vi "acquireAndDetectTest.vi"() -> ()   [LabVIEW 2024]
uses:
  elements/black-squircle-dropdown.ctl
  toolkit/modelParameters.ctl
  elements/black-squircle-ring.ctl
  <vilib>/userDefined/High Color/IMAQdx.ctl
  <vilib>/Utility/error.llb/DialogType.ctl
  <vilib>/vision/driver/NI_Vision_Acquisition_Software.lvlib
  <resource>/objmgr/imaqdx.rc
  toolkit/transformCv.lvclass
panel:
  out "error status":string
  in  "update model":bool
  in  "res":T1 caption="Resolution:" items=["160x120 YUY2 30.00fps", "320x180 YUY2 30.00fps", "320x240 YUY2 30.00fps", "424x240 YUY2 30.00fps", "640x360 MJPG 30.00fps", "640x360 YUY2 30.00fps", "640x480 MJPG 30.00fps", "640x480 YUY2 30.00fps", "848x480 MJPG 30.00fps", "960x540 MJPG 30.00fps", "1280x720 MJPG 30.00fps"]
  in  "pause":bool
  in  "model params":T2={"conf"=0.25, "iou"=0.5, "model w"=1280, "model h"=736, "img w "=1280, "img h"=736} caption="Model Parameters"
  in  "classes":path caption="Class Definition Path"
  in  "model":path caption="Model Path"
  in  "cpu/gpu":enum32{"Item 0", "Item 1"}(radio)=enum."Item 1"
  in  "play":bool
  in  "cam":T3 caption="Camera:"
  out "img":T4(plugin-control)
  out "tot detect":i32 caption="Total Detections"
  # "Transform-CV Acquire and Detect Demo v1.0.0"
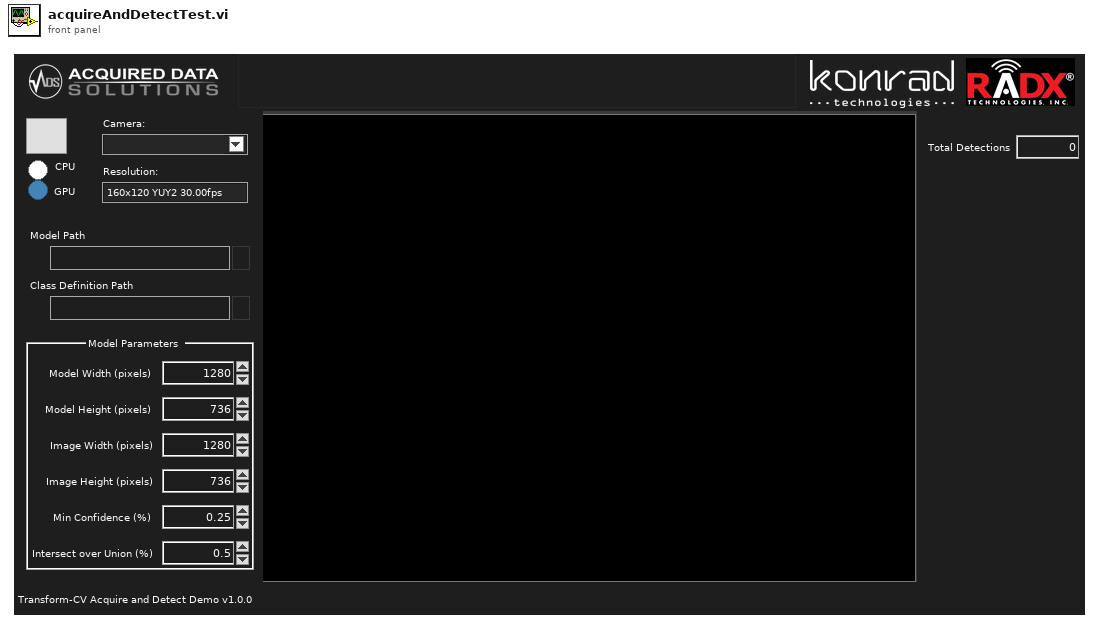
[diagram p1: front panel]
types:
  T1 = typedef "black-squircle-ring.ctl" = u16
  T2 = typedef "transformCv.lvclass/modelParameters.ctl" = cluster{"conf":dbl, "iou":dbl, "model w":i32, "model h":i32, "img w ":i32, "img h":i32}
  T3 = typedef "black-squircle-dropdown.ctl" = string
  T4 = typedef "IMAQ Image.ctl" = refnum<image>
  T5 = typedef "IMAQdx.ctl" = refnum<k21>
  T6 = cluster{"Left":i32, "Top":i32, "Right":i32, "Bottom":i32}
  T7 = typedef "transformCv.lvclass/rectangularDetectedObject.ctl" = cluster{"x1":sgl, "y1":sgl, "x2":sgl, "y2":sgl, "conf":sgl, "cls":i32}
  T8 = typedef "DialogType.ctl" = u16
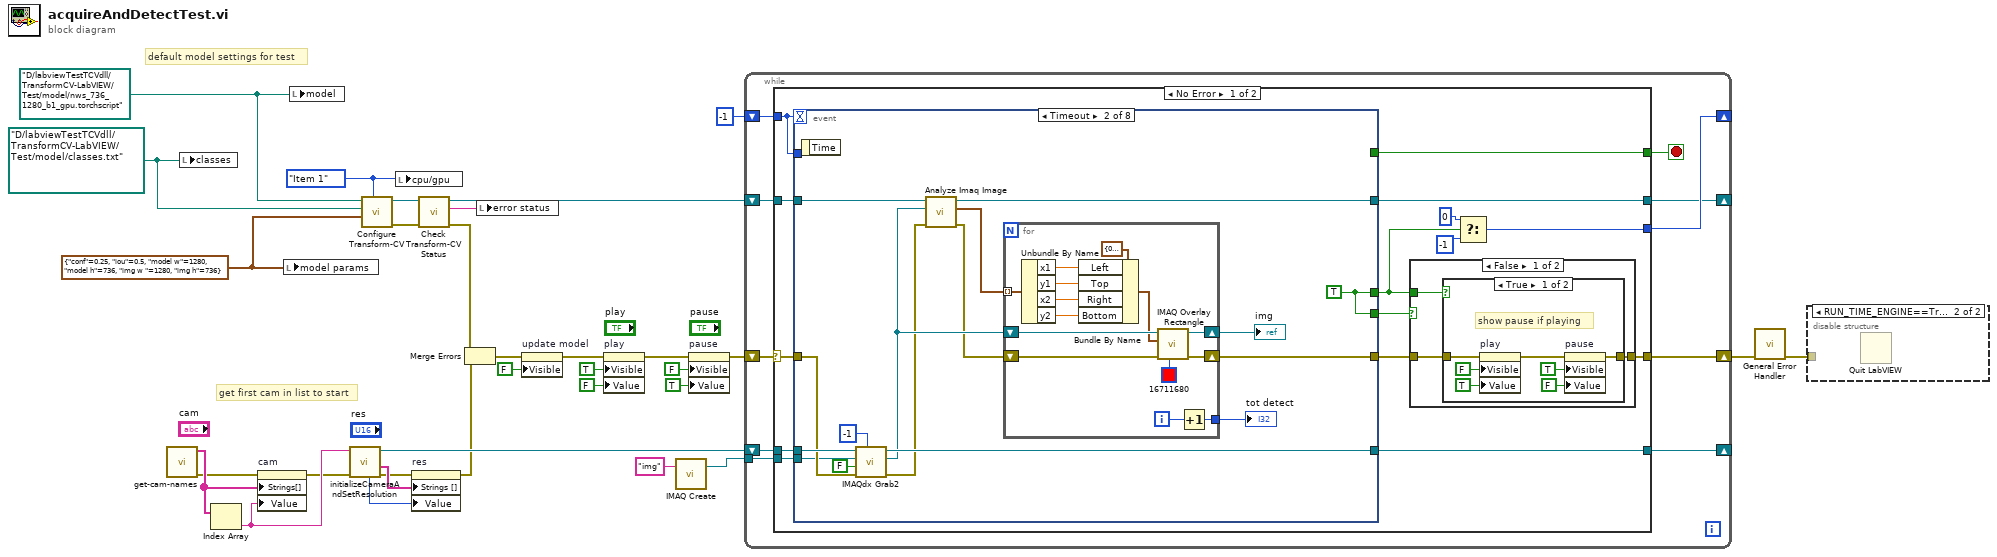
[diagram p0: block diagram]
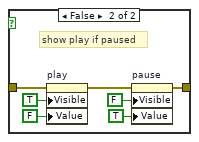
[diagram p3: hidden frame]
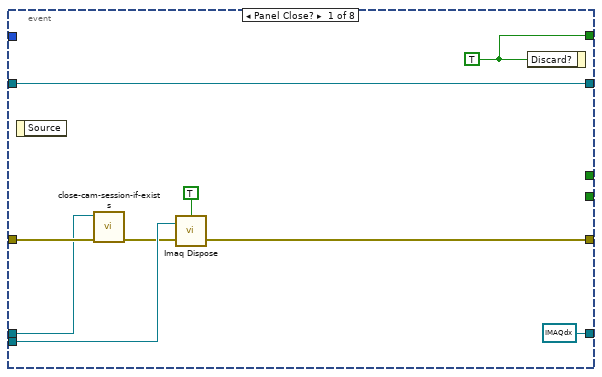
[diagram p5: hidden frame]
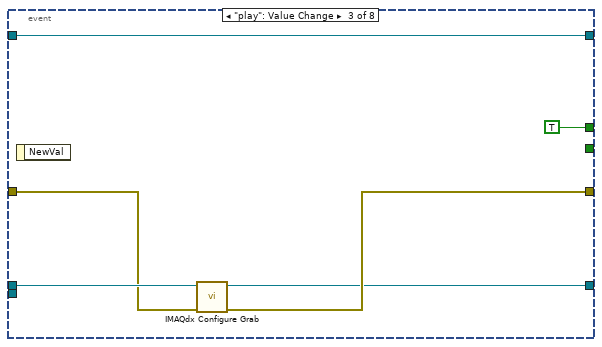
[diagram p6: hidden frame]
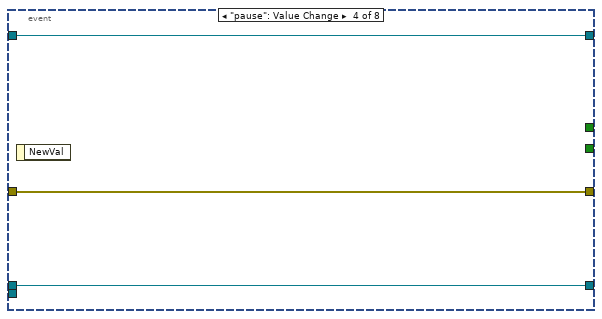
[diagram p7: hidden frame]
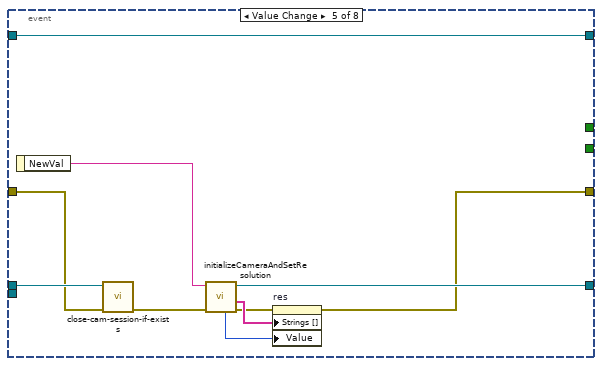
[diagram p8: hidden frame]
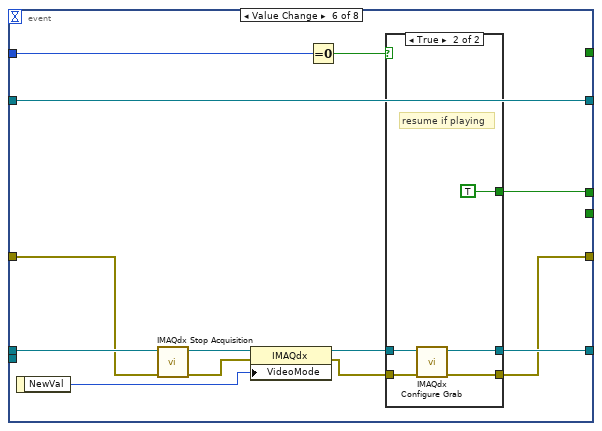
[diagram p9: hidden frame]
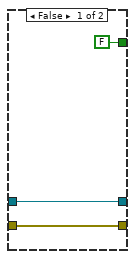
[diagram p10: hidden frame]
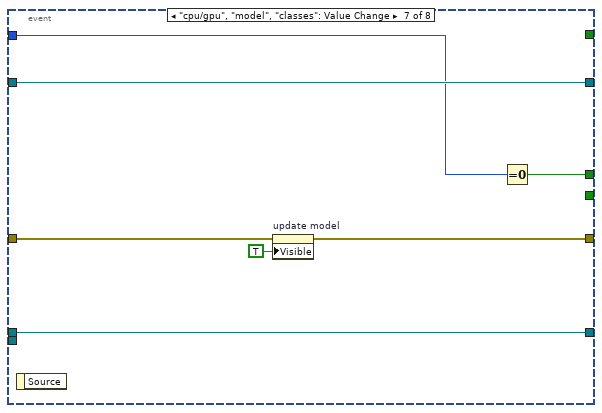
[diagram p11: hidden frame]
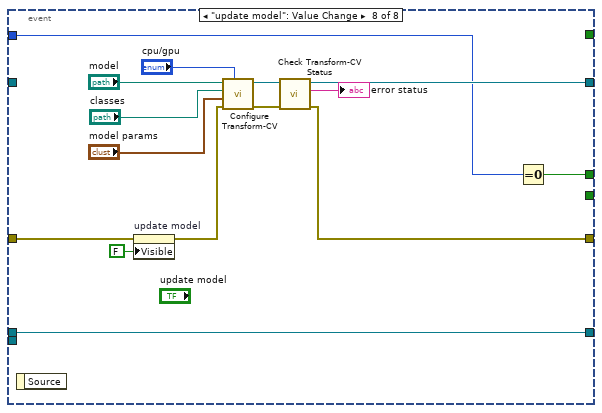
[diagram p12: hidden frame]
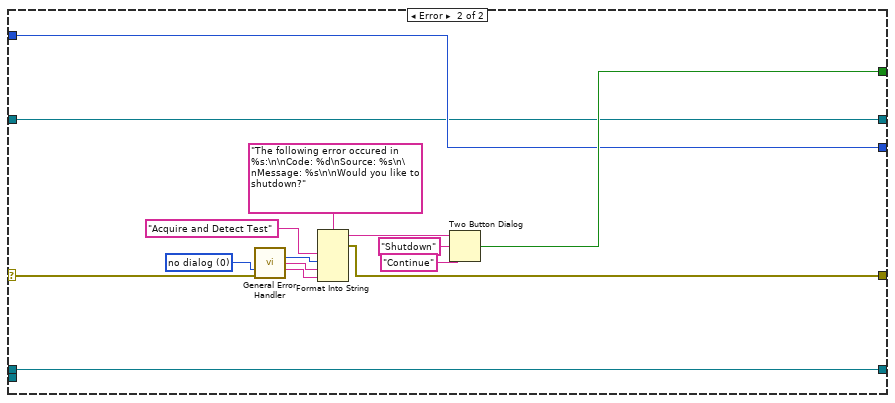
[diagram p13: hidden frame]
diagram:
  w8 = enum32{"Item 0", "Item 1"}."Item 1" ("cpu/gpu")
  w11 = T2 {"conf"=0.25, "iou"=0.5, "model w"=1280, "model h"=736, "img w "=1280, "img h"=736} ("model params")
  w12 = path "D:/labviewTestTCVdll/TransformCV-LabVIEW/Test/model/classes.txt" ("model")
  w13 = path "D:/labviewTestTCVdll/TransformCV-LabVIEW/Test/model/nws_736_1280_b1_gpu.torchscript" ("model")
  # "get first cam in list to start"
  # "default model settings for test"
  n1 = call "get-cam-names.vi"() -> ("error out"=w14:errorcluster, "cam names"=w25:string[])  [unwired: 10 in]
  n2 = local write "classes"(w12) -> ()
  n3 = Index Array(array=w25) -> (element=w24:string)  [unwired: 1 in]
  n4 = property on="cam" class="CmbBox (strict)"(error in=w14, "Strings[]"=w25, "Value"=w24) -> (error out=w23:errorcluster)  [unwired: 1 in, 1 out]
  n5 = local write "model params"(w11) -> ()
  n6 = local write "model"(w13) -> ()
  n7 = call "initializeCameraAndSetResolution.vi"("error in"=w23, "seesion in"=w24) -> ("error out"=w20:errorcluster, "mode names"=w22:string[], "session out"=w19:T5, "current mode"=w21:u32)  [unwired: 5 in, 1 out]
  n8 = call "Configure Transform-CV.vi"("cpu/gpu"=w8, "model params"=w11, "classes"=w12, "model"=w13) -> ("error out"=w6:errorcluster, "transformCvToolkit out"=w7:refnum<class "transformCv.lvclass">)  [unwired: 5 in, 1 out]
  n9 = local write "cpu/gpu"(w8) -> ()
  n10 = property on="res" class="Ring (strict)"(error in=w20, "Strings []"=w22, "Value"=w21) -> (error out=w10:errorcluster)  [unwired: 1 in, 1 out]
  n11 = call "Check Transform-CV Status.vi"("error in (no error)"=w6, "transformCv in"=w7) -> ("error out"=w5:errorcluster, "status"=w3:string, "transformCv out"=w4:refnum<class "transformCv.lvclass">)  [unwired: 7 in]
  n12 = Merge Errors(w5, w10) -> (w9:errorcluster)
  n13 = local write "error status"(w3) -> ()
  n14 = property on="update model" class="Bool"(error in=w9, "Visible"=FALSE) -> (error out=w16:errorcluster)  [unwired: 1 in, 1 out]
  n15 = property on="play" class="Bool (strict)"(error in=w16, "Visible"=TRUE, "Value"=FALSE ("play")) -> (error out=w30:errorcluster)  [unwired: 1 in, 1 out]
  n16 = call "IMAQ Create"("Image Name"="img") -> ("New Image"=w17:T4)  [unwired: 4 in, 1 out]
  n17 = property on="pause" class="Bool (strict)"(error in=w30, "Visible"=FALSE, "Value"=TRUE ("Visible")) -> (error out=w31:errorcluster)  [unwired: 1 in, 1 out]
  n18 = while {
    shift-right: [w42] -> w2
    shift-left: w31 -> [w41]
    shift-right: [w38] -> _
    shift-left: -1 -> [w39]
    shift-right: [w36] -> _
    shift-left: w19 -> [w37]
    tunnel: w17 -> [w35]
    shift-right: [w33] -> _
    shift-left: w4 -> [w34]
    stop <- w40 stop-if-true
    n19 = case shown="No Error" w41 {
      selector: w41 -> [w57 w183]
      tunnel: [w51 w181] -> w42
      tunnel: [w56 w182] -> w40
      tunnel: w39 -> [w45 w179]
      tunnel: [w53 w179] -> w38
      tunnel: w37 -> [w48 w178]
      tunnel: [w47 w178] -> w36
      tunnel: w35 -> [w46 _]
      tunnel: w34 -> [w44 w177]
      tunnel: [w43 w177] -> w33
      frame No Error {
        n20 = event shown="[1] Timeout" {
          selector: _ -> [_ _ _ _ _ _ _ _]
          dyn-events: _ -> [_ _ _ _ _ _ _ _]
          timeout: w45 -> [_ _ _ _ _ _ _ _]
          tunnel: w57 -> [w78 w96 w118 w123 w127 w143 w159 w166]
          tunnel: [w84 _ _ _ _ _ _ _] -> w56
          tunnel: [w81 w88 w117 w123 w125 w136 w158 w164] -> w52
          tunnel: [_ w100 TRUE ("s") _ _ w135 w155 w162] -> w50
          tunnel: [_ w100 _ _ _ _ _ _] -> w49
          tunnel: w48 -> [w76 w97 w119 w122 w128 w145 w160 w172]
          tunnel: [T5 refnum ("session out") w95 w116 w122 w132 w137 w160 w172] -> w47
          tunnel: w46 -> [w80 w94 _ _ _ _ _ _]
          tunnel: w45 -> [_ _ _ _ _ w141 w156 w163]
          tunnel: w44 -> [w83 w93 w115 w121 w124 w134 w161 _]
          tunnel: [w83 w86 w115 w121 w124 w134 w161 w174] -> w43
          event Panel Close? {
            w84 = TRUE ("Discard?")
            n21 = event-data() -> ()  [unwired: 1 in, 1 out]
            n22 = call "close-cam-session-if-exists.vi"("error in (no error)"=w78, "cam in"=w76) -> ("error out"=w77:errorcluster)  [unwired: 9 in]
            n23 = call "Imaq Dispose"("All Images? (No)"=TRUE, "Image"=w80, "error in (no error)"=w77) -> ("error out"=w81:errorcluster)  [unwired: 3 in]
            n24 = event-data("Discard?"=w84) -> ()  [unwired: 1 in, 1 out]
          }
          event Timeout {
            w100 = TRUE ("s")
            n25 = event-data() -> ()  [unwired: 1 in, 1 out]
            n26 = call <vilib>:"IMAQdx Grab2.vi"("Timeout (ms)"=-1, "error in"=w96, "Wait for Next Buffer? (Yes)"=FALSE, "Image In"=w94, "Session In"=w97) -> ("error out"=w91:errorcluster, "Image Out"=w92:T4, "Session Out"=w95:T5)  [unwired: 3 in, 1 out]
            n27 = call "Analyze Imaq Image.vi"("error in (no error)"=w91, "imaq image ref"=w92, "transformCv in"=w93) -> ("error out"=w89:errorcluster, "objects"=w90:T7[], "transformCv out"=w86:refnum<class "transformCv.lvclass">)  [unwired: 6 in]
            n28 = for {
              tunnel: w90 -> [w112] mode=indexing
              shift-right: [w104] -> w87
              shift-left: w92 -> [w114]
              shift-right: [w103] -> w88
              shift-left: w89 -> [w113]
              tunnel: [w101] -> w85
              i -> [w102]
              n29 = Unbundle By Name(w112) -> ("x1"=w110:sgl, "y1"=w109:sgl, "x2"=w108:sgl, "y2"=w107:sgl)
              n30 = Bundle By Name(cluster=T6 {"Left"=0, "Top"=0, "Right"=0, "Bottom"=0} ("Rectangle"), "Left"=w110, "Top"=w109, "Right"=w108, "Bottom"=w107) -> (w106:T6)
              n31 = call "IMAQ Overlay Rectangle"("Color"=u32 16711680, "error in (no error)"=w113, "Rectangle"=w106, "Image"=w114) -> ("error out"=w103:errorcluster, "Image Out"=w104:T4)  [unwired: 6 in]
              n32 = Increment(x=w102) -> (x+1=w101:i32)
            }
            "img" <- w87
            "tot detect" <- w85
          }
          event "play": Value Change {
            n33 = event-data() -> ()  [unwired: 1 in, 1 out]
            n34 = call <vilib>:"IMAQdx Configure Grab.vi"("error in"=w118, "Session In"=w119) -> ("error out"=w117:errorcluster, "Session Out"=w116:T5)  [unwired: 8 in]
          }
          event "pause": Value Change {
            n35 = event-data() -> ()  [unwired: 1 in, 1 out]
          }
          event Value Change {
            n36 = event-data() -> ("NewVal"=w133:T3)  [unwired: 1 in]
            n37 = call "close-cam-session-if-exists.vi"("error in (no error)"=w127, "cam in"=w128) -> ("error out"=w126:errorcluster)  [unwired: 9 in]
            n38 = call "initializeCameraAndSetResolution.vi"("error in"=w126, "seesion in"=w133) -> ("error out"=w130:errorcluster, "mode names"=w131:string[], "session out"=w132:T5, "current mode"=w129:u32)  [unwired: 5 in, 1 out]
            n39 = property on="res" class="Ring (strict)"(error in=w130, "Strings []"=w131, "Value"=w129) -> (error out=w125:errorcluster)  [unwired: 1 in, 1 out]
          }
          event Value Change {
            n40 = event-data() -> ("NewVal"=w146:T1)  [unwired: 1 in]
            n41 = call <vilib>:"IMAQdx Stop Acquisition.vi"("error in"=w143, "Session In"=w145) -> ("error out"=w142:errorcluster, "Session Out"=w144:T5)  [unwired: 8 in]
            n42 = property class="IMAQdx"(reference=w144, error in=w142, "VideoMode"=w146) -> (reference out=w139:T5, error out=w138:errorcluster)
            n43 = Equal To 0?(x=w141) -> (x = 0?=w140:bool)
            n44 = case shown="True" w140 {
              tunnel: w139 -> [w148 w154]
              tunnel: w138 -> [w147 w153]
              tunnel: [w148 w152] -> w137
              tunnel: [w147 w151] -> w136
              tunnel: [FALSE ("s") TRUE ("s")] -> w135
              frame False {
              }
              frame True {
                # "resume if playing"
                n45 = call <vilib>:"IMAQdx Configure Grab.vi"("error in"=w153, "Session In"=w154) -> ("error out"=w151:errorcluster, "Session Out"=w152:T5)  [unwired: 8 in]
              }
            }
          }
          event "cpu/gpu", "model", "classes": Value Change {
            n46 = event-data() -> ()  [unwired: 1 in, 1 out]
            n47 = property on="update model" class="Bool"(error in=w159, "Visible"=TRUE) -> (error out=w158:errorcluster)  [unwired: 1 in, 1 out]
            n48 = Equal To 0?(x=w156) -> (x = 0?=w155:bool)
          }
          event "update model": Value Change {
            n49 = event-data() -> ()  [unwired: 1 in, 1 out]
            n50 = property on="update model" class="Bool"(error in=w166, "Visible"=FALSE) -> (error out=w165:errorcluster)  [unwired: 1 in, 1 out]
            n51 = call "Configure Transform-CV.vi"("cpu/gpu"="cpu/gpu", "error in (no error)"=w165, "model params"="model params", "classes"="classes", "model"="model") -> ("error out"=w176:errorcluster, "transformCvToolkit out"=w175:refnum<class "transformCv.lvclass">)  [unwired: 4 in, 1 out]
            n52 = call "Check Transform-CV Status.vi"("error in (no error)"=w176, "transformCv in"=w175) -> ("error out"=w164:errorcluster, "status"=→"error status":string, "transformCv out"=w174:refnum<class "transformCv.lvclass">)  [unwired: 7 in]
            n53 = Equal To 0?(x=w163) -> (x = 0?=w162:bool)
          }
        }
        n54 = case shown="False" w49 {
          tunnel: w52 -> [w60 w75]
          tunnel: [w59 w75] -> w51
          tunnel: w50 -> [w58 _]
          frame False {
            n55 = case shown="True" w58 {
              tunnel: w60 -> [w62 w69]
              tunnel: [w61 w68] -> w59
              frame True {
                # "show pause if playing"
                n56 = property on="play" class="Bool (strict)"(error in=w62, "Visible"=FALSE, "Value"=TRUE ("play")) -> (error out=w64:errorcluster)  [unwired: 1 in, 1 out]
                n57 = property on="pause" class="Bool (strict)"(error in=w64, "Visible"=TRUE, "Value"=FALSE ("Visible")) -> (error out=w61:errorcluster)  [unwired: 1 in, 1 out]
              }
              frame False {
                # "show play if paused"
                n58 = property on="play" class="Bool (strict)"(error in=w69, "Visible"=TRUE, "Value"=FALSE ("play")) -> (error out=w71:errorcluster)  [unwired: 1 in, 1 out]
                n59 = property on="pause" class="Bool (strict)"(error in=w71, "Visible"=FALSE, "Value"=TRUE ("Visible")) -> (error out=w68:errorcluster)  [unwired: 1 in, 1 out]
              }
            }
          }
          frame True {
            # "don't waste time on update if running continuous acquisition"
          }
        }
        n60 = Select(t=0, s=w50, f=-1) -> (s? t:f=w53:i32)
      }
      frame Error {
        w191 = T8 0 items=["no dialog", "OK message", "continue or stop message", "OK message + warnings", "continue/stop + warnings"] ("type of dialog (OK msg:1)")
        n61 = call <vilib>:"General Error Handler.vi"("type of dialog (OK msg:1)"=w191, "error in (no error)"=w183) -> ("code out"=w184:i32, "source out"=w186:string, "message"=w187:string)  [unwired: 9 in, 2 out]
        n62 = Format Into String(format string="The following error occured in %s:\n\nCode: %d\nSource: %s\n\nMessage: %s\n\nWould you like to shutdown?", "Acquire and Detect Test" ("input 1"), w184, w186, w187) -> (resulting string=w188:string, error out=w181:errorcluster)  [unwired: 2 in]
        n63 = Two Button Dialog(message=w188, 1:"Continue" ("F button name (\"Cancel\")"), 2:"Shutdown" ("T button name (\"OK\")")) -> (T button?=w182:bool)
      }
    }
  }
  n64 = call <vilib>:"General Error Handler.vi"("error in (no error)"=w2) -> ("error out"=w1:errorcluster)  [unwired: 10 in, 4 out]
  n65 = disable-structure shown="RUN_TIME_ENGINE==True" {
    disable-tunnel: w1 -> [_ _]
    frame condition #0 (active) {
    }
    frame condition #1 {
      n66 = Quit LabVIEW() -> ()  [unwired: 1 in]
    }
  }
